vi "Set Number.vi"(8 "error in (no error)":errorcluster, 10 "Numeric":dbl, 11 "Callback Consumer in":refnum<class "Callback Consumer.lvclass">) -> (0 "error out":errorcluster, 3 "Callback Consumer out":refnum<class "Callback Consumer.lvclass">)   [LabVIEW 2012, in "Callback Consumer.lvclass"]
uses:
  Callback Consumer.lvclass
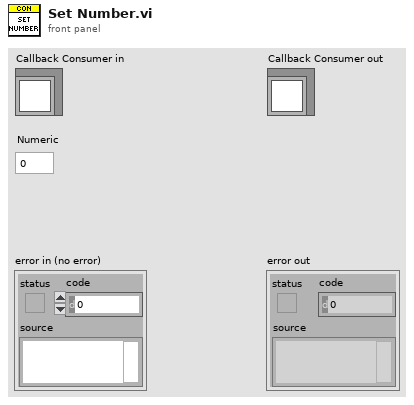
[diagram p1: front panel]
types:
  T1 = typedef "Callback Consumer.lvclass/Ref Data.ctl" = cluster{"Numeric":dbl}
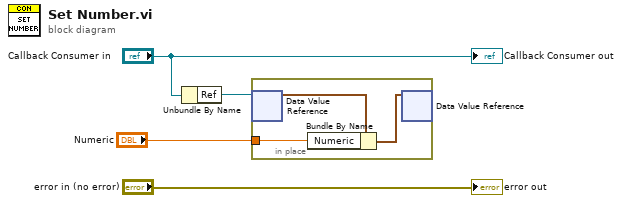
[diagram p0: block diagram]
diagram:
  n1 = Unbundle By Name("Callback Consumer in") -> ("Ref"=w3:refnum<data-value>)
  n2 = in-place {
    in-place-border: "Numeric" -> [w5]
    n3 = in-place-dvr #1(w3) -> (w7:T1)  [unwired: 1 out]
    n4 = Bundle By Name(cluster=w7, "Numeric"=w5) -> (w6:T1)
    n5 = in-place-dvr #1(w6) -> ()  [unwired: 2 out]
  }
  "error out" <- "error in (no error)"
  "Callback Consumer out" <- "Callback Consumer in"
